vi "Open Phys Chan Property.vi"(0 "session in":refnum<k21>, 5 "physical channel":refnum<k21>="$DefaultPhysChans", 7 "property in":refnum<k21>, 11 "error in (no error)":errorcluster) -> (4 "session out":refnum<k21>, 8 "property out":refnum<k21>, 15 "error out":errorcluster)   [LabVIEW 2020, in "SLSC.lvlib"]
doc: "Opens a reference to a physical channel property. This allows the application to programmatically get information about the property at run time."
uses:
  <vilib>/SLSC/SLSC.lvlib
  nislsclvapi.dll
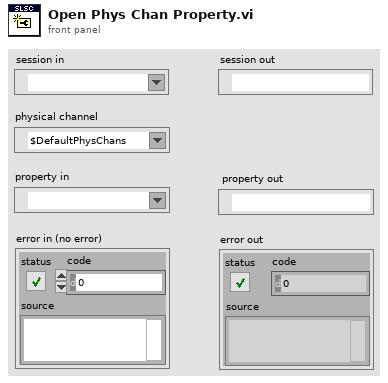
[diagram p1: front panel]
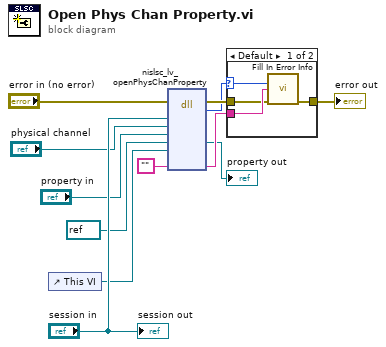
[diagram p0: block diagram]
diagram:
  n1 = control-ref of="This VI"() -> (w2:refnum<vi>)
  n2 = dll-call lib="nislsclvapi.*" fn="nislsc_lv_openPhysChanProperty"(error in="error in (no error)", "session"="session in", "physChan"="physical channel", "propertyIn"="property in", "propertyRefObjOut"=refnum<k21> refnum ("property out"), "lvAppRef"=w2, "extendedErrorInfo"="") -> (error out=w9:errorcluster, "return type"=w8:i32, "propertyRefObjOut"=→"property out":refnum<k21>, "extendedErrorInfo"=w10:string)  [unwired: 8 in, 1 out]
  n3 = case shown="Default" w8 {
    selector: w8 -> [w16 _]
    tunnel: w10 -> [w15 _]
    tunnel: w9 -> [w14 w17]
    tunnel: [w13 w17] -> w7
    frame Default {
      n4 = call <vilib>:"Fill In Error Info.vi"("status code"=w16, "extended error info"=w15, "error in"=w14) -> ("error out"=w13:errorcluster)  [unwired: 12 in]
    }
    frame 0 {
    }
  }
  "error out" <- w7
  "session out" <- "session in"
